vi "read_csv.vi"(8 "error in":errorcluster, 11 "file path (dialog if empty)":path) -> (0 "error out":errorcluster, 3 "Degrees arr(lon, lat)":dbl[][](array[numeric]) format="%#.9g")   [LabVIEW 2020]
uses:
  <vilib>/Utility/file.llb/Read Delimited Spreadsheet (DBL).vi
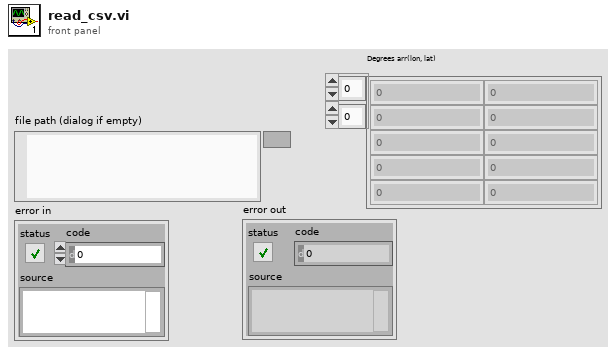
[diagram p1: front panel]
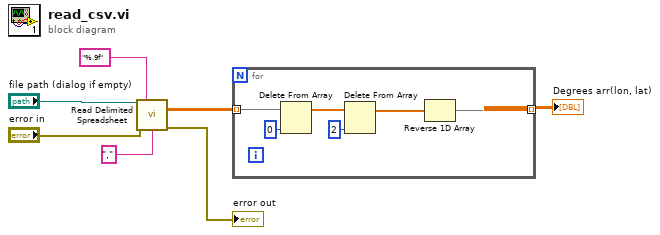
[diagram p0: block diagram]
diagram:
  n1 = call-poly <vilib>:"Read Delimited Spreadsheet.vi"("file path (dialog if empty)"="file path (dialog if empty)", "format (%.3f)"="%.9f", "error in (no error)"="error in", "delimiter (\\t)"="," ("delimiter (\\t)")) -> ("all rows"=w2:dbl[][], "error out"=→"error out":errorcluster)  [unwired: 6 in, 4 out]
  n2 = for {
    tunnel: w2 -> [w13] mode=indexing
    tunnel: [w8] -> w1 mode=indexing
    n3 = Delete From Array(array=w13, index=0) -> (array with subset deleted=w11:dbl[])  [unwired: 1 in, 1 out]
    n4 = Delete From Array(array=w11, index=2) -> (array with subset deleted=w9:dbl[])  [unwired: 1 in, 1 out]
    n5 = Reverse 1D Array(array=w9) -> (reversed array=w8:dbl[])
  }
  "Degrees arr(lon, lat)" <- w1
